vi "Filter_Table_Test.vi"() -> ()   [LabVIEW 2025, in "Table_Filtering.lvlib"]
uses:
  Table_Filtering.lvlib
  <vilib>/Utility/miscctls.llb/LVRowAndColumnUnsignedTypeDef.ctl
  e1f20763-3153-4008-8b66-4090a748bc05.vi
  <vilib>/Array/Sort 2D Array - Pop Stack.vi
  <vilib>/Array/Sort 2D Array - Push Stack.vi
panel:
  in  "Filter String":string="Protocol == UDP AND Length > 0.7 OR Source == 192.168.1.1"
  in  "Sort by":u16(ring) items=["Packet_Number", "Timestamp", "Source", "Destination", "Protocol", "Length", "Data"]
  in  "Headers":string[](array[string])=["Packet_Number", "Timestamp", "Source", "Destination", "Protocol", "Length", "Data"]
  in  "Pause":bool
  out "Table Control":string[][](table)
  in  "stop":bool
  in  "Visible Columns":bool[](array[boolean])
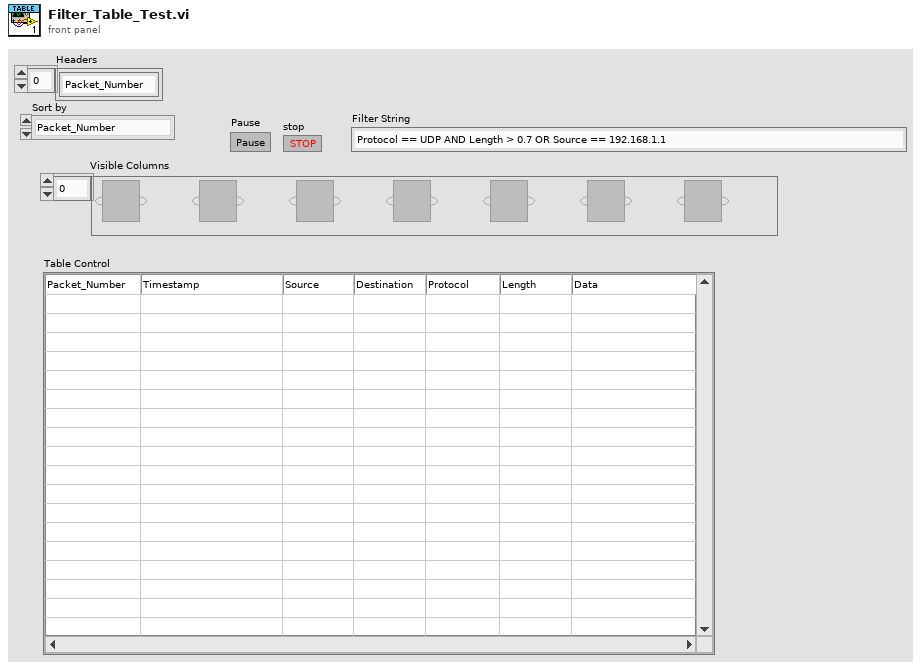
[diagram p1: front panel]
types:
  T1 = typedef "LVRowAndColumnUnsignedTypeDef.ctl" = cluster{"Row":u32, "Column":u32}
  T2 = cluster{"FIELD":string, "OPERATOR":string, "VALUE":string}[]
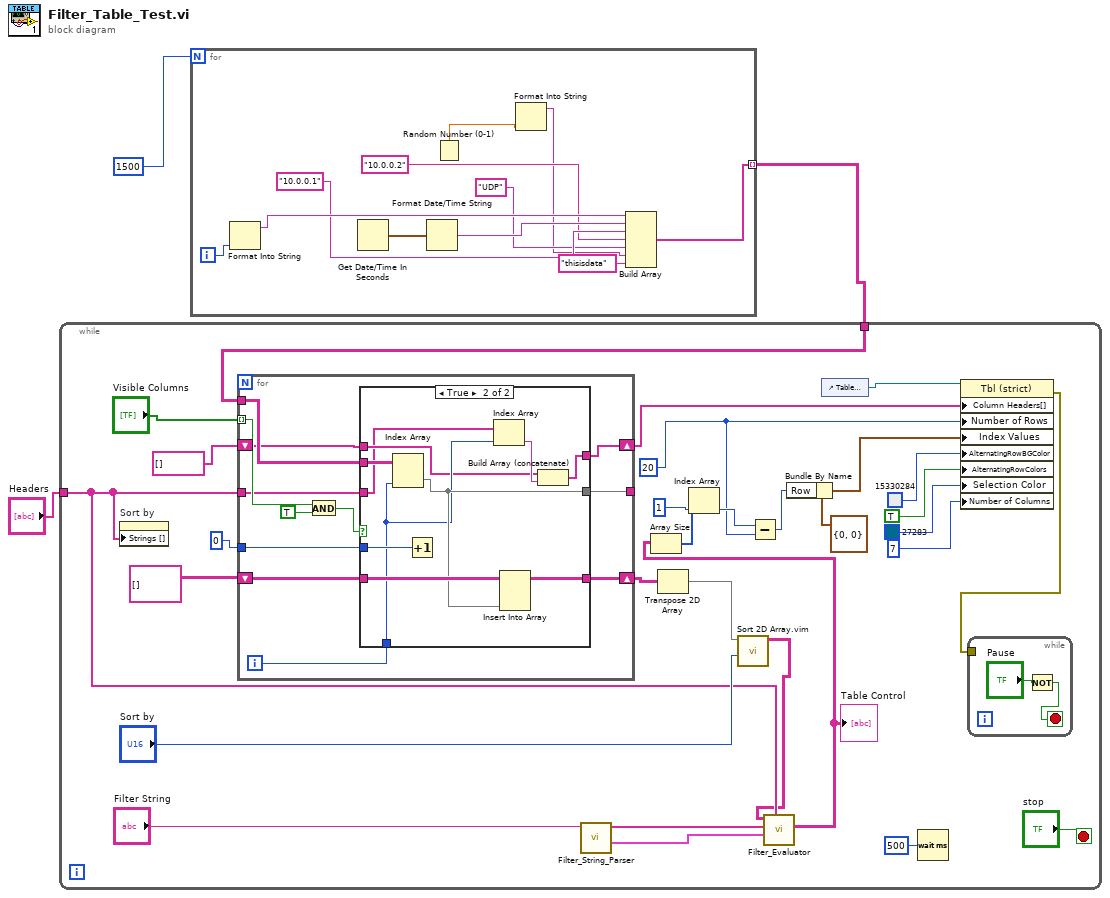
[diagram p0: block diagram]
diagram:
  n1 = for {
    N: 1500 ("Numeric") -> [_]
    tunnel: [w14] -> w2 mode=indexing
    i -> [w13]
    n2 = Format Into String(w13) -> (resulting string=w12:string)  [unwired: 3 in, 1 out]
    n3 = Get Date/Time In Seconds() -> (seconds since 1Jan1904=w11:timestamp)
    n4 = Format Date/Time String(seconds (now)=w11) -> (date/time string=w10:string)  [unwired: 2 in]
    n5 = Random Number (0-1)() -> (number: 0 to 1=w6:dbl)
    n6 = Format Into String(w6) -> (resulting string=w5:string)  [unwired: 3 in, 1 out]
    n7 = Build Array(w12, w10, "10.0.0.1", "10.0.0.2", "UDP", w5, "thisisdata" ("element")) -> (w14:string[])
  }
  n8 = while {
    tunnel: w2 -> [w44]
    tunnel: "Headers" -> [w17]
    stop <- "stop" stop-if-true
    w35 = u32 20 ("Number of Rows")
    n9 = property on="Sort by" class="Ring (strict)"("Strings []"=w17) -> ()  [unwired: 2 in, 2 out]
    n10 = for {
      tunnel: "Visible Columns" -> [w56] mode=indexing
      tunnel: w44 -> [w58]
      tunnel: [w53] -> _
      shift-right: [w52] -> w39
      shift-left: string[][] [] ("array") -> [w54]
      tunnel: 0 -> [w50]
      shift-right: [w48] -> w41
      shift-left: string[] [] -> [w49]
      tunnel: w17 -> [w47]
      i -> [w57]
      n11 = And(x=w56, y=TRUE) -> (x .and. y?=w51:bool)
      n12 = case shown="True" w51 {
        tunnel: w58 -> [_ w70]
        tunnel: w57 -> [_ w65]
        tunnel: w54 -> [w60 w69]
        tunnel: [_ w68] -> w53
        tunnel: [w60 w67] -> w52
        tunnel: w50 -> [_ w66]
        tunnel: [w59 w64] -> w48
        tunnel: w49 -> [w59 w62]
        tunnel: w47 -> [_ w61]
        frame False {
        }
        frame True {
          n13 = Index Array(array=w70, index (col)=w65) -> (element=w68:string[])  [unwired: 1 in]
          n14 = Increment(x=w66) -> ()  [unwired: 1 out]
          n15 = Index Array(array=w61, index=w65) -> (element=w63:string)
          n16 = Insert Into Array(array=w69, new element=w68) -> (w67:string[][])  [unwired: 2 in]
          n17 = Build Array (concatenate)(w62, w63) -> (w64:string[])
        }
      }
    }
    n18 = call "Filter_String_Parser.vi"("Filter String"="Filter String") -> ("Comparators"=w19:T2, "Boolean Connectors"=w18:string[])  [unwired: 9 in]
    n19 = Transpose 2D Array(2D array=w39) -> (transposed array=w31:string[][])
    n20 = call "Sort 2D Array.vim"("index"="Sort by", "2D array"=w31) -> ("sorted 2D array"=w16:string[][])  [unwired: 8 in, 1 out]
    n21 = call "Filter_Evaluator.vi"("Headers"=w17, "Comparators"=w19, "Boolean Connectors"=w18, "Prefiltered Data"=w16) -> ("Filtered Array"=w15:string[][])  [unwired: 6 in, 1 out]
    "Table Control" <- w15
    n22 = Array Size(array=w15) -> (size(s)=w38:i32[])
    n23 = Index Array(array=w38, index=1) -> (element=w36:i32)
    n24 = Subtract(x=w36, y=w35) -> (x-y=w34:u32)
    n25 = Bundle By Name(cluster=T1 {"Row"=0, "Column"=0} ("Index Values"), "Row"=w34) -> (w33:T1)
    n26 = control-ref of="Table Control"() -> (w24:refnum<vi>)
    n27 = Wait (ms)(milliseconds to wait=u32 500) -> ()  [unwired: 1 out]
    n28 = property on="Property Node" class="Tbl (strict)"(reference=w24, "Column Headers[]"=w41, "Number of Rows"=w35, "Index Values"=w33, "AlternatingRowBGColor"=u32 15330284 ("Alternate Row Background Color"), "AlternatingRowColors"=TRUE ("Alternating Row Colors"), "Selection Color"=u32 27283, "Number of Columns"=u32 7) -> (error out=w25:errorcluster)  [unwired: 1 in, 1 out]
    n29 = while {
      tunnel: w25 -> [_]
      stop <- w45 stop-if-true
      n30 = Not(x="Pause") -> (.not. x?=w45:bool)
    }
  }
